vi "Check.vi"(8 "error in (no error)":errorcluster, 11 "Blacklist in":refnum<class "Blacklist.lvclass">) -> (0 "error out":errorcluster, 1 "Reject?":bool, 3 "Blacklist out":refnum<class "Blacklist.lvclass">)   [LabVIEW 2014, in "lvbuildsecurity.lvlib" / "Blacklist.lvclass"]
uses:
  Blacklist.lvclass
  <vilib>/Utility/traverseref.llb/TRef TravTarget.ctl
  Blacklist.lvclass/Blacklist.ctl
  <vilib>/Utility/traverseref.llb/VI Scripting - Traverse.lvlib
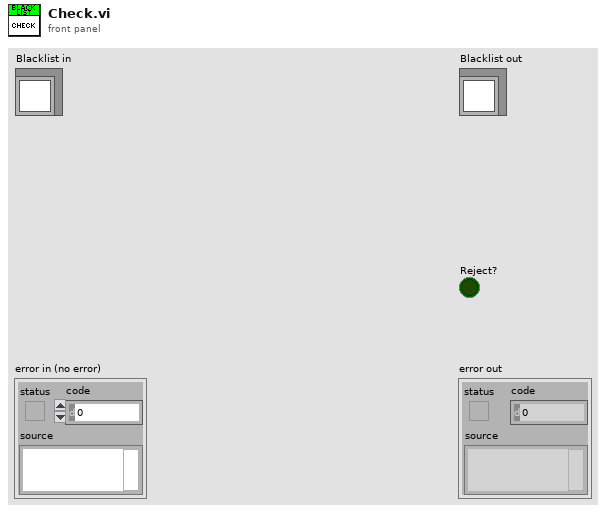
[diagram p1: front panel]
types:
  T1 = typedef "TRef TravTarget.ctl" = enum16{"FP", "BD", "Other"}
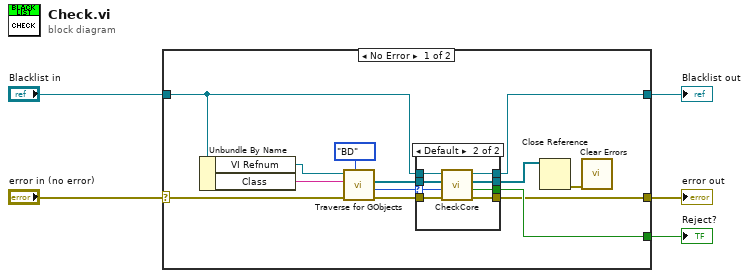
[diagram p0: block diagram]
diagram:
  n1 = case shown="No Error" "error in (no error)" {
    selector: "error in (no error)" -> [w16 w31]
    tunnel: [w11 w31] -> w4
    tunnel: [w8 w30] -> w2
    tunnel: "Blacklist in" -> [w9 w30]
    tunnel: [w12 _] -> w1
    frame No Error {
      n2 = Unbundle By Name(w9) -> ("VI Refnum"=w6:refnum<vi>, "Class"=w17:string)
      n3 = call <vilib>:"Traverse for GObjects.vi"("Traverse Target"=TRef_TravTarget."BD", "error in (no error)"=w16, "Class Name"=w17, "VI Refnum"=w6) -> ("error out"=w15:errorcluster, "# of Refs"=w7:i32, "References"=w14:refnum<vi>[])  [unwired: 4 in, 1 out]
      n4 = case shown="Default" w7 {
        selector: w7 -> [_ w22]
        tunnel: w15 -> [w19 w29]
        tunnel: w14 -> [w20 w28]
        tunnel: [w20 w27] -> w13
        tunnel: [_ w26] -> w12
        tunnel: [w19 w25] -> w11
        tunnel: [w21 w24] -> w8
        tunnel: w9 -> [w21 w23]
        frame 0 {
        }
        frame Default {
          n5 = call-dynamic "CheckCore.vi"("error in (no error)"=w29, "# of Refs"=w22, "References"=w28, "Blacklist in"=w23) -> ("error out"=w25:errorcluster, "Reject?"=w26:bool, "dup References"=w27:refnum<vi>[], "Blacklist out"=w24:refnum<class "Blacklist.lvclass">)  [unwired: 4 in]
        }
      }
      n6 = Close Reference(reference=w13) -> (error out=w10:errorcluster)  [unwired: 1 in]
      n7 = call <vilib>:"Clear Errors.vi"("error in (no error)"=w10) -> ()  [unwired: 5 in, 2 out]
    }
    frame Error {
    }
  }
  "error out" <- w4
  "Blacklist out" <- w2
  "Reject?" <- w1
